vi "getSelected.vi"(9 "Amp":dbl[](array[numeric]), 10 "Weight":i32[](array[numeric]), 11 "Predict":i32[](array[numeric])) -> (3 "selected":i32)   [LabVIEW 2014]
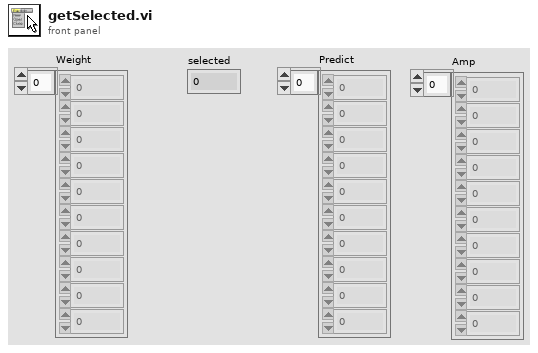
[diagram p1: front panel]
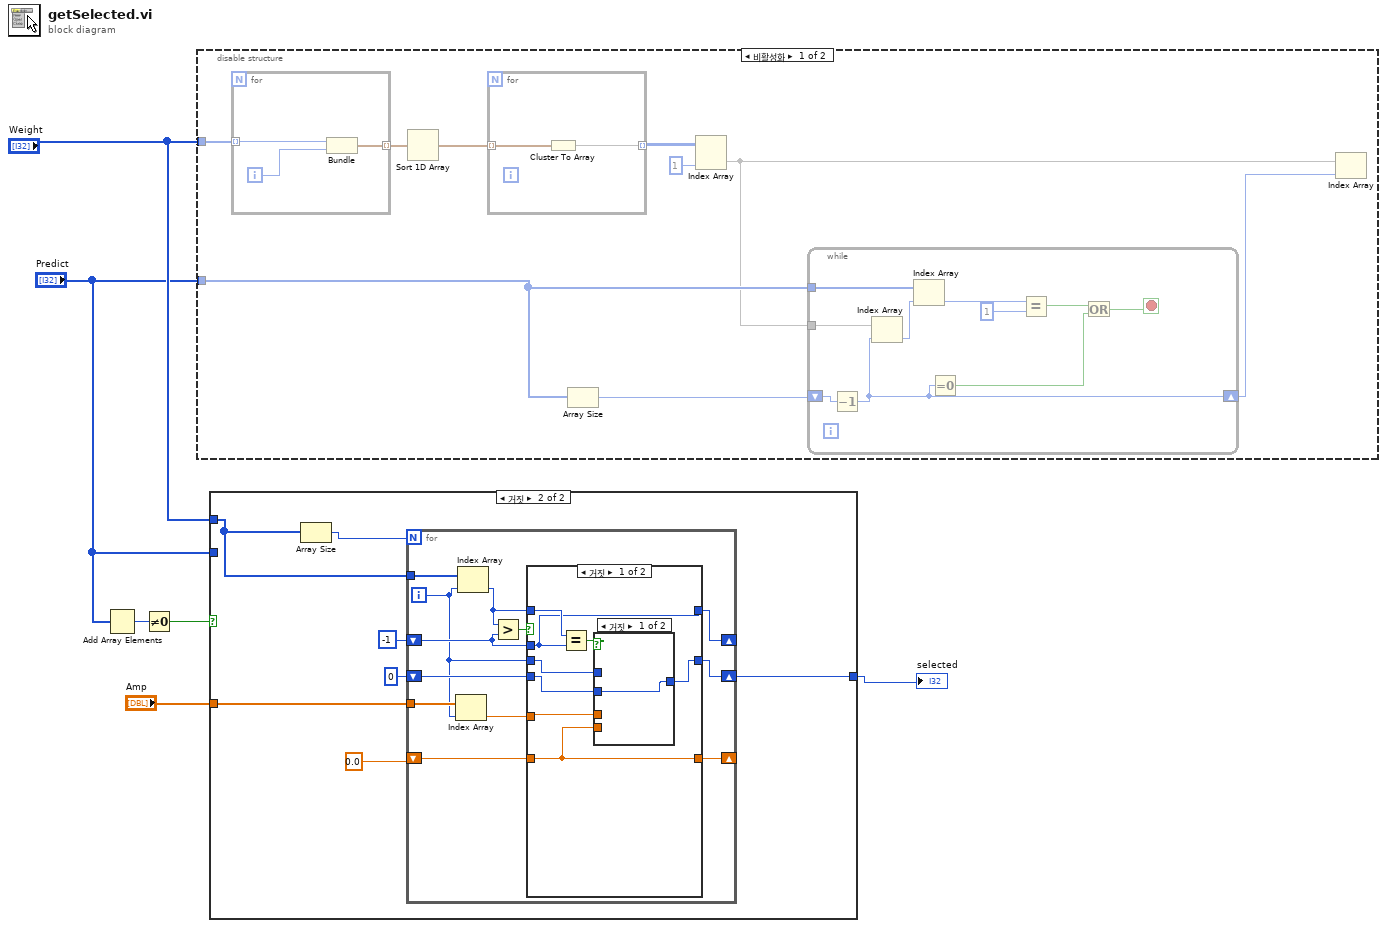
[diagram p0: block diagram]
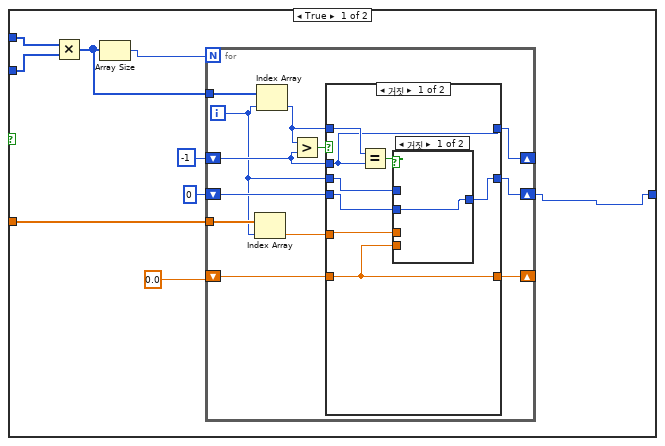
[diagram p2: hidden frame]
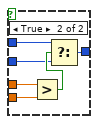
[diagram p3: hidden frame]
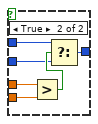
[diagram p5: hidden frame]
diagram:
  n1 = Add Array Elements(numeric array="Predict") -> (sum=w3:i32)
  n2 = Not Equal To 0?(x=w3) -> (x != 0?=w2:bool)
  n3 = disable-structure shown="비활성화" {
    disable-tunnel: "Weight" -> [w15 _]
    disable-tunnel: "Predict" -> [w14 _]
    frame Disabled {
      n4 = for {
        tunnel: w15 -> [w20] mode=indexing
        tunnel: [w19] -> w13 mode=indexing
        i -> [w18]
        n5 = Bundle("Numeric"=w20, w18) -> (w19:cluster{"Numeric":i32, i32})  [unwired: 1 in]
      }
      n6 = Sort 1D Array(array=w13) -> (sorted array=w12:cluster{"Numeric":i32, i32}[])
      n7 = for {
        tunnel: w12 -> [w17] mode=indexing
        tunnel: [w16] -> w11 mode=indexing
        n8 = Cluster To Array(cluster=w17) -> (array=w16:i32[])
      }
      n9 = Array Size(array=w14) -> (size(s)=w9:i32)
      n10 = Index Array(array=w11, index (col)=1 ("index")) -> (element=w8:i32[])  [unwired: 1 in]
      n11 = while {
        tunnel: w14 -> [w24]
        shift-right: [w26] -> w7
        shift-left: w9 -> [w28]
        tunnel: w8 -> [w25]
        stop <- w30 stop-if-true
        n12 = Decrement(x=w28) -> (x-1=w26:i32)
        n13 = Index Array(array=w25, index=w26) -> (element=w23:i32)
        n14 = Index Array(array=w24, index=w23) -> (element=w22:i32)
        n15 = Equal To 0?(x=w26) -> (x = 0?=w27:bool)
        n16 = Equal?(x=w22, y=1) -> (x = y?=w29:bool)
        n17 = Or(x=w29, y=w27) -> (x .or. y?=w30:bool)
      }
      n18 = Index Array(array=w8, index=w7) -> ()  [unwired: 1 out]
    }
    frame Enabled {
    }
  }
  n19 = case shown="거짓" w2 {
    tunnel: "Weight" -> [w39 w71]
    tunnel: "Predict" -> [w38 _]
    tunnel: "Amp" -> [w33 w73]
    tunnel: [w31 w70] -> w4
    frame True {
      n20 = Multiply(x=w39, y=w38) -> (x*y=w37:i32[])
      n21 = Array Size(array=w37) -> (size(s)=w36:i32)
      n22 = for {
        N: w36 -> [_]
        tunnel: w37 -> [w51]
        shift-right: [w49] -> _
        shift-left: -1 -> [w47]
        shift-right: [w45] -> w31
        shift-left: 0 -> [w46]
        tunnel: w33 -> [w44]
        shift-right: [w42] -> _
        shift-left: 0.0 -> [w40]
        i -> [w43]
        n23 = Index Array(array=w44, index=w43) -> (element=w41:dbl)
        n24 = Index Array(array=w51, index=w43) -> (element=w48:i32)
        n25 = Greater?(x=w48, y=w47) -> (0:w50:bool)
        n26 = case shown="거짓" w50 {
          tunnel: [w58 w69] -> w49
          tunnel: w48 -> [w59 w69]
          tunnel: w47 -> [w58 _]
          tunnel: w46 -> [w52 _]
          tunnel: [w54 w68] -> w45
          tunnel: w43 -> [w53 w68]
          tunnel: [w56 w67] -> w42
          tunnel: w41 -> [w55 w67]
          tunnel: w40 -> [w56 _]
          frame False {
            n27 = Equal?(x=w59, y=w58) -> (x = y?=w57:bool)
            n28 = case shown="거짓" w57 {
              tunnel: w56 -> [_ w66]
              tunnel: w55 -> [_ w65]
              tunnel: [w60 w64] -> w54
              tunnel: w53 -> [_ w62]
              tunnel: w52 -> [w60 w61]
              frame False {
              }
              frame True {
                n29 = Greater?(x=w65, y=w66) -> (0:w63:bool)
                n30 = Select(t=w62, s=w63, f=w61) -> (s? t:f=w64:i32)
              }
            }
          }
          frame True {
          }
        }
      }
    }
    frame False {
      n31 = Array Size(array=w71) -> (size(s)=w76:i32)
      n32 = for {
        N: w76 -> [_]
        tunnel: w71 -> [w88]
        shift-right: [w86] -> _
        shift-left: -1 -> [w84]
        shift-right: [w82] -> w70
        shift-left: 0 -> [w83]
        tunnel: w73 -> [w81]
        shift-right: [w79] -> _
        shift-left: 0.0 -> [w77]
        i -> [w80]
        n33 = Index Array(array=w81, index=w80) -> (element=w78:dbl)
        n34 = Index Array(array=w88, index=w80) -> (element=w85:i32)
        n35 = Greater?(x=w85, y=w84) -> (0:w87:bool)
        n36 = case shown="거짓" w87 {
          tunnel: [w95 w106] -> w86
          tunnel: w85 -> [w96 w106]
          tunnel: w84 -> [w95 _]
          tunnel: w83 -> [w89 _]
          tunnel: [w91 w105] -> w82
          tunnel: w80 -> [w90 w105]
          tunnel: [w93 w104] -> w79
          tunnel: w78 -> [w92 w104]
          tunnel: w77 -> [w93 _]
          frame False {
            n37 = Equal?(x=w96, y=w95) -> (x = y?=w94:bool)
            n38 = case shown="거짓" w94 {
              tunnel: w93 -> [_ w103]
              tunnel: w92 -> [_ w102]
              tunnel: [w97 w101] -> w91
              tunnel: w90 -> [_ w99]
              tunnel: w89 -> [w97 w98]
              frame False {
              }
              frame True {
                n39 = Greater?(x=w102, y=w103) -> (0:w100:bool)
                n40 = Select(t=w99, s=w100, f=w98) -> (s? t:f=w101:i32)
              }
            }
          }
          frame True {
          }
        }
      }
    }
  }
  "selected" <- w4
